vi "MCS_VariableGap_161102.vi"() -> ()   [LabVIEW 2010]
panel:
  out "Number of Step":dbl
  out "Current Step":dbl
  out "Status":string
  out "error out":errorcluster
  out "Stage 3 Position (um)":i32
  out "Stage 2 Position (um)":i32
  out "Stage 1 Position (um)":i32
  in  "Desired Gap (um)":i32
  in  "Home Detection Direction":T1(ring)
  in  "error in (no error)":errorcluster
  in  "MCS System Locator":string
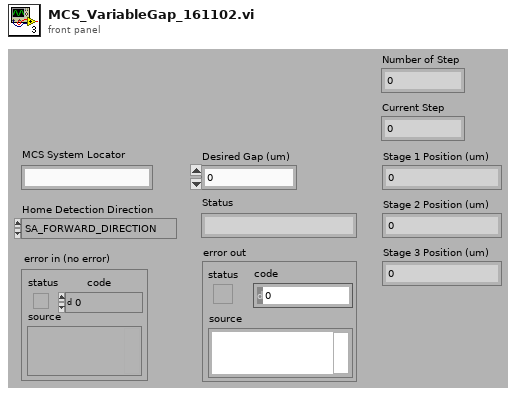
[diagram p1: front panel]
types:
  T1 = enum32{"SA_FORWARD_DIRECTION", "SA_BACKWARD_DIRECTION", "SA_FORWARD_BACKWARD_DIRECTION", "SA_BACKWARD_FORWARD_DIRECTION"}
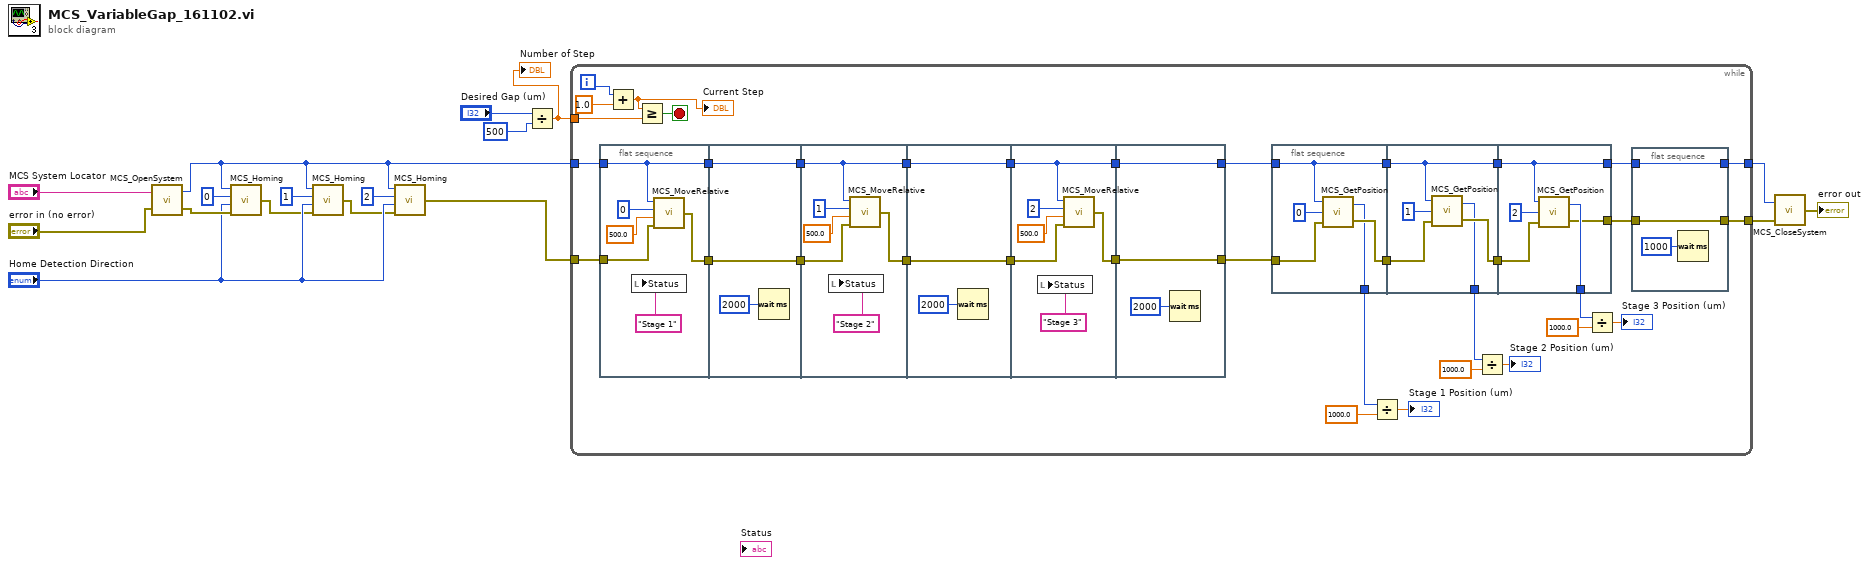
[diagram p0: block diagram]
diagram:
  n1 = call "MCS_OpenSystem.vi"("error in (no error)"="error in (no error)", "MCS System Locator"="MCS System Locator") -> ("error out"=w14:errorcluster, "System Index Out"=w8:u32)
  n2 = call "MCS_Homing.vi"("error in (no error)"=w14, "Direction"="Home Detection Direction", "Channel Index In"=u32 0, "System Index In"=w8) -> ("error out"=w10:errorcluster)
  n3 = call "MCS_Homing.vi"("error in (no error)"=w10, "Direction"="Home Detection Direction", "Channel Index In"=u32 1, "System Index In"=w8) -> ("error out"=w9:errorcluster)
  n4 = call "MCS_Homing.vi"("error in (no error)"=w9, "Direction"="Home Detection Direction", "Channel Index In"=u32 2, "System Index In"=w8) -> ("error out"=w7:errorcluster)
  n5 = Divide(x="Desired Gap (um)", y=500) -> (x/y=w3:dbl)
  "Number of Step" <- w3
  n6 = while {
    tunnel: w8 -> [w39]
    tunnel: w7 -> [w38]
    tunnel: w3 -> [w26]
    tunnel: [w24] -> w2
    tunnel: [w22] -> w1
    i -> [w20]
    stop <- w18 stop-if-true
    n7 = flat-sequence {
      tunnel: [w57] -> w49
      tunnel: w39 -> [w56]
      tunnel: [w56] -> w48
      tunnel: w38 -> [w55]
      tunnel: w49 -> [w62]
      tunnel: [w62] -> w47
      tunnel: w48 -> [w61]
      tunnel: [w61] -> w46
      tunnel: w47 -> [w66]
      tunnel: [w65] -> w45
      tunnel: w46 -> [w64]
      tunnel: [w64] -> w44
      tunnel: w45 -> [w71]
      tunnel: [w71] -> w43
      tunnel: w44 -> [w70]
      tunnel: [w70] -> w42
      tunnel: w43 -> [w75]
      tunnel: w42 -> [w73]
      tunnel: [w74] -> w41
      tunnel: [w73] -> w40
      tunnel: [w79] -> w28
      tunnel: [w80] -> w27
      tunnel: w41 -> [w80]
      tunnel: w40 -> [w79]
      frame #0 {
        n8 = local write "Status"("Stage 1" ("Status")) -> ()
        n9 = call "MCS_MoveRelative.vi"("error in (no error)"=w55, "Moving Distance (um)"=500.0, "Channel Index In"=u32 0, "System Index In"=w56) -> ("error out"=w57:errorcluster)
      }
      frame #1 {
        n10 = Wait (ms)(milliseconds to wait=u32 2000) -> ()  [unwired: 1 out]
      }
      frame #2 {
        n11 = local write "Status"("Stage 2" ("Status")) -> ()
        n12 = call "MCS_MoveRelative.vi"("error in (no error)"=w66, "Moving Distance (um)"=500.0, "Channel Index In"=u32 1, "System Index In"=w64) -> ("error out"=w65:errorcluster)
      }
      frame #3 {
        n13 = Wait (ms)(milliseconds to wait=u32 2000) -> ()  [unwired: 1 out]
      }
      frame #4 {
        n14 = local write "Status"("Stage 3" ("Status")) -> ()
        n15 = call "MCS_MoveRelative.vi"("error in (no error)"=w75, "Moving Distance (um)"=500.0, "Channel Index In"=u32 2, "System Index In"=w73) -> ("error out"=w74:errorcluster)
      }
      frame #5 {
        n16 = Wait (ms)(milliseconds to wait=u32 2000) -> ()  [unwired: 1 out]
      }
    }
    n17 = Add(x=w20, y=1.0) -> (x+y=w19:dbl)
    "Current Step" <- w19
    n18 = Greater Or Equal?(x=w19, y=w26) -> (x >= y?=w18:bool)
    n19 = flat-sequence {
      tunnel: w28 -> [w87]
      tunnel: [w87] -> w53
      tunnel: w27 -> [w86]
      tunnel: [w85] -> w52
      tunnel: [w84] -> w30
      tunnel: w53 -> [w89]
      tunnel: [w89] -> w51
      tunnel: w52 -> [w92]
      tunnel: [w91] -> w50
      tunnel: [w90] -> w32
      tunnel: [w95] -> w25
      tunnel: w51 -> [w95]
      tunnel: w50 -> [w97]
      tunnel: [w96] -> w35
      tunnel: [w94] -> w23
      frame #0 {
        n20 = call "MCS_GetPosition.vi"("error in (no error)"=w86, "Channel Index In"=u32 0, "System Index In"=w87) -> ("error out"=w85:errorcluster, "Position"=w84:i32)
      }
      frame #1 {
        n21 = call "MCS_GetPosition.vi"("error in (no error)"=w92, "Channel Index In"=u32 1, "System Index In"=w89) -> ("error out"=w91:errorcluster, "Position"=w90:i32)
      }
      frame #2 {
        n22 = call "MCS_GetPosition.vi"("error in (no error)"=w97, "Channel Index In"=u32 2, "System Index In"=w95) -> ("error out"=w94:errorcluster, "Position"=w96:i32)
      }
    }
    n23 = Divide(x=w30, y=1000.0) -> (x/y=→"Stage 1 Position (um)":dbl)
    n24 = Divide(x=w32, y=1000.0) -> (x/y=→"Stage 2 Position (um)":dbl)
    n25 = Divide(x=w35, y=1000.0) -> (x/y=→"Stage 3 Position (um)":dbl)
    n26 = flat-sequence {
      tunnel: w25 -> [w82]
      tunnel: [w82] -> w24
      tunnel: [w81] -> w22
      tunnel: w23 -> [w81]
      frame #0 {
        n27 = Wait (ms)(milliseconds to wait=u32 1000) -> ()  [unwired: 1 out]
      }
    }
  }
  n28 = call "MCS_CloseSystem.vi"("error in (no error)"=w1, "System Index In"=w2) -> ("error out"=→"error out":errorcluster)
